vi "Set subscription map.vi"(8 "error in (no error)":errorcluster {"code" format="Error %.0f"}, 10 "subscription map":refnum<data-value>, 11 "NATS Client in":refnum<class "NATS Client.lvclass">) -> (0 "error out":errorcluster {"code" format="Error %.0f"}, 3 "NATS Client out":refnum<class "NATS Client.lvclass">)   [LabVIEW 2020, in "NATS Client.lvlib" / "NATS Client.lvclass"]
uses:
  NATS Client.lvclass
  NATS Subscription/NATS Subscription.lvclass
  NATS Client.lvclass/NATS Client.ctl
  Subscription Map.ctl
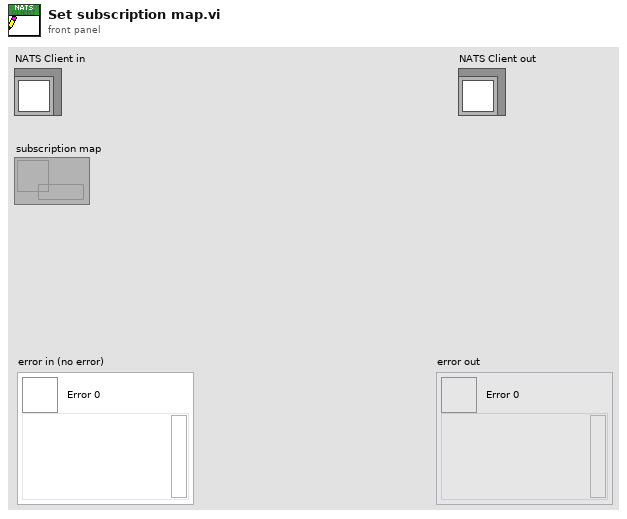
[diagram p1: front panel]
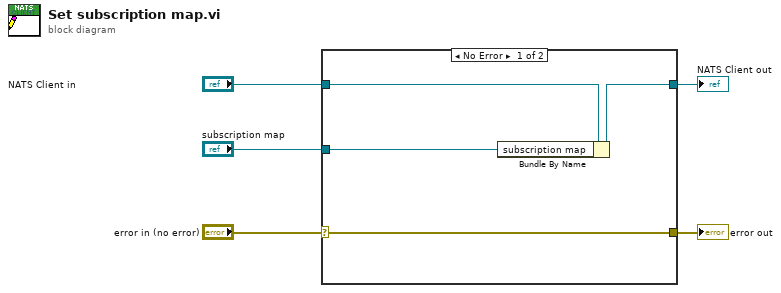
[diagram p0: block diagram]
diagram:
  n1 = case shown="No Error" "error in (no error)" {
    selector: "error in (no error)" -> [w9 w10]
    tunnel: [w9 w10] -> w4
    tunnel: [w7 w11] -> w2
    tunnel: "NATS Client in" -> [w8 w11]
    tunnel: "subscription map" -> [w6 _]
    frame No Error {
      n2 = Bundle By Name(cluster=w8, "subscription map"=w6) -> (w7:refnum<class "NATS Client.lvclass">)
    }
    frame Error {
    }
  }
  "error out" <- w4
  "NATS Client out" <- w2
